vi "Food Order.vi"() -> ()   [LabVIEW 2023]
panel:
  in  "Back":bool
  in  "Food Order 2":bool
  out "Order Details":string
  in  "Food Order":bool
  out "2D Picture 2":picture
  out "Food Items":T1(array[cluster])
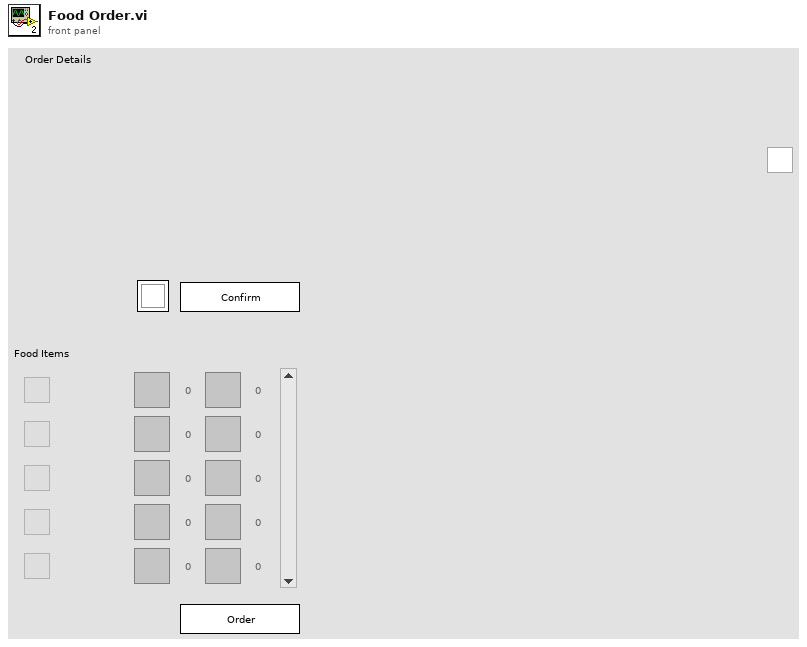
[diagram p1: front panel]
types:
  T1 = cluster{"2D Picture 3":picture, "Name":string, "Add Button":bool, "Remove Button":bool, "Numeric":u32, "Numeric 2":u32}[]
  T2 = cluster{"2D Picture 3":picture, "Name":string, "Add Button":bool, "Remove Button":bool, "Numeric":u32, "Numeric 2":u32}
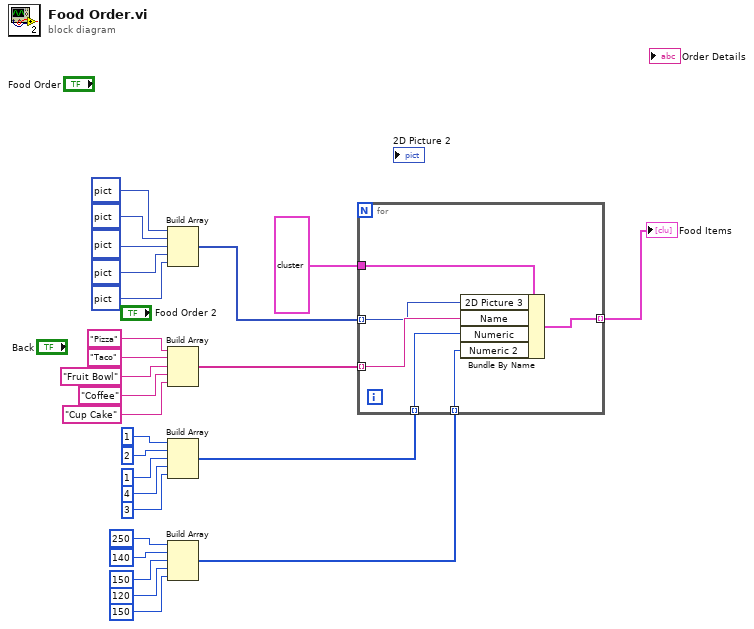
[diagram p0: block diagram]
diagram:
  n1 = Build Array(picture bytes[2136] ("2D Picture"), picture bytes[2136] ("2D Picture"), picture bytes[2808] ("2D Picture"), picture bytes[2058] ("2D Picture"), picture bytes[2217] ("2D Picture")) -> (w14:picture[])
  n2 = Build Array("Pizza" ("Name"), "Taco" ("Name"), "Fruit Bowl" ("Name"), "Coffee" ("Name"), "Cup Cake" ("Name")) -> (w15:string[])
  n3 = Build Array(u32 1 ("Numeric"), u32 2 ("Numeric"), u32 1 ("Numeric"), u32 4 ("Numeric"), u32 3 ("Numeric")) -> (w7:u32[])
  n4 = Build Array(u32 250 ("Numeric"), u32 140 ("Numeric"), u32 150 ("Numeric"), u32 120 ("Numeric"), u32 150 ("Numeric")) -> (w1:u32[])
  n5 = for {
    tunnel: T2 {"2D Picture 3"=bytes[0], "Name"="", "Add Button"=FALSE, "Remove Button"=FALSE, "Numeric"=0, "Numeric 2"=0} ("Food Item") -> [w32]
    tunnel: w15 -> [w31] mode=indexing
    tunnel: w14 -> [w30] mode=indexing
    tunnel: [w29] -> w13 mode=indexing
    tunnel: w7 -> [w28] mode=indexing
    tunnel: w1 -> [w27] mode=indexing
    n6 = Bundle By Name(cluster=w32, "2D Picture 3"=w30, "Name"=w31, "Numeric"=w28, "Numeric 2"=w27) -> (w29:T2)
  }
  "Food Items" <- w13
